vi "Initialize Results Tree.vi"(8 "error in (no error)":errorcluster, 10 "Pane width":u32, 11 "TreeControl in":refnum<vi>) -> (0 "error out":errorcluster, 3 "reference out":refnum<vi>)   [LabVIEW 2020, in "Execution UI V2.lvclass"]
uses:
  Execution UI V2.lvclass
  Execution UI V2.lvclass/Execution UI V2.ctl
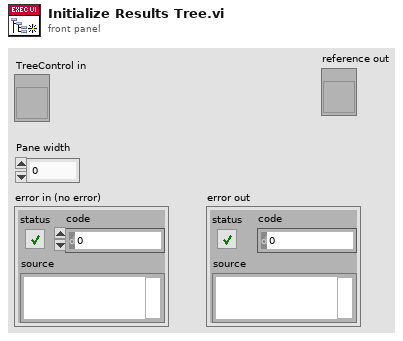
[diagram p1: front panel]
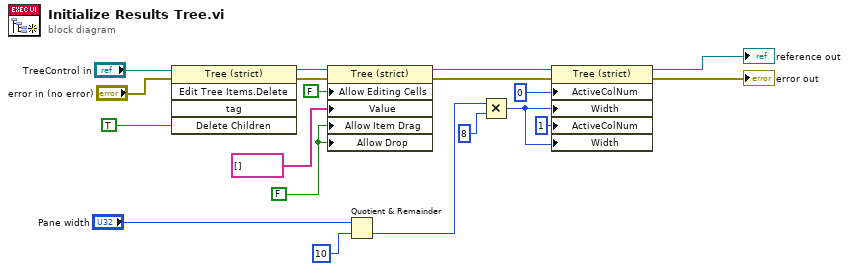
[diagram p0: block diagram]
diagram:
  w1 = FALSE ("Drag/Drop:Allow Dragging")
  n1 = invoke on="Invoke Node" class="Tree (strict)" method="Edit Tree Items.Delete"(reference="TreeControl in", error in="error in (no error)", "Delete Children"=TRUE ("Delete Children?")) -> (reference out=w14:refnum<vi>, error out=w16:errorcluster)  [unwired: 2 in, 3 out]
  n2 = property class="Tree (strict)"(reference=w14, error in=w16, "Allow Editing Cells"=FALSE, "Value"=string[] [], "Allow Item Drag"=w1, "Allow Drop"=w1) -> (reference out=w6:refnum<vi>, error out=w5:errorcluster)
  n3 = Quotient & Remainder(x="Pane width", y=u32 10) -> (floor(x/y)=w10:u32)  [unwired: 1 out]
  n4 = Multiply(x=w10, y=u32 8) -> (x*y=w7:u32)
  n5 = property on="Property Node" class="Tree (strict)"(reference=w6, error in=w5, "ActiveColNum"=0 ("Active Cell:Active Column Number"), "Width"=w7, "ActiveColNum"=1 ("Active Cell:Active Column Number"), "Width"=w7) -> (reference out=→"reference out":refnum<vi>, error out=→"error out":errorcluster)
